vi "LeCroy - Transfer External To Ext Or Ext10.vi"(4 "Trigger Level 2":dbl, 6 "Trigger Level":dbl, 8 "error in (no error)":errorcluster, 10 "Trigger Source With External":u16, 11 "VISA resource name":refnum<visa-resource-name>) -> (0 "error out":errorcluster, 2 "Trigger Source With Ext/Ext10":u16, 3 "VISA resource name out":refnum<visa-resource-name>)   [LabVIEW 8.6]
doc: "This is function which transfer Eternal trigger source to Ext and Ext10. Another trigger source are retained in same state. Transfer External source to Ext and Ext10 is make with compare trigger level. When is trigger level greater than 400 mV (for WaveSurfer 500 mV), than External trigger source is transfer to the Ext10, else is transfer to the Ext."
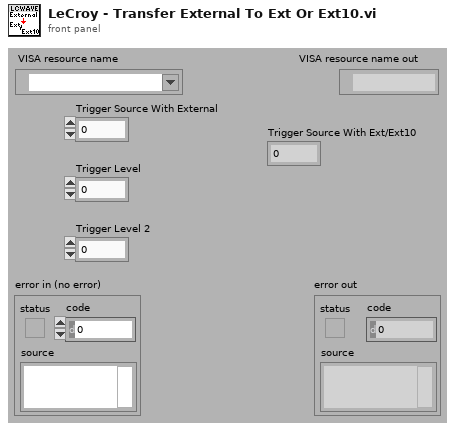
[diagram p1: front panel]
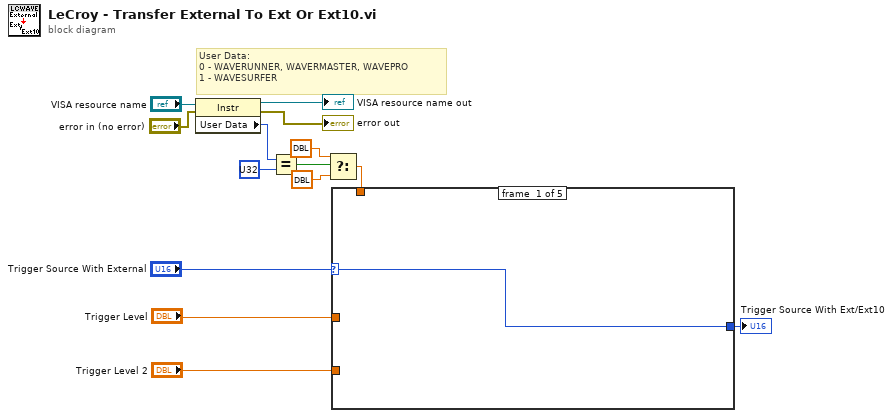
[diagram p0: block diagram]
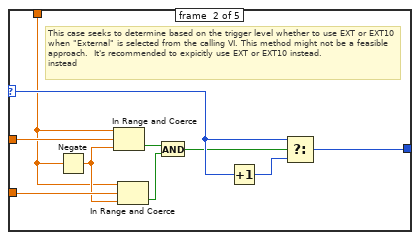
[diagram p2: hidden frame]
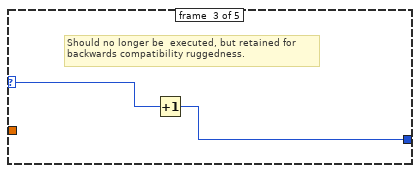
[diagram p3: hidden frame]
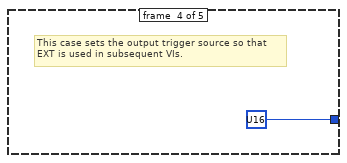
[diagram p4: hidden frame]
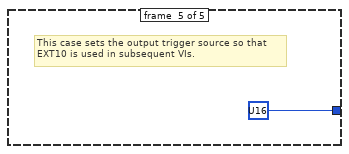
[diagram p5: hidden frame]
diagram:
  # "User Data:\n0 - WAVERUNNER, WAVERMASTER, WAVEPRO\n1 - WAVESURFER"
  n1 = property on="Property Node" class="Instr"(reference="VISA resource name", error in="error in (no error)") -> (reference out=→"VISA resource name out":refnum<visa-resource-name>, error out=→"error out":errorcluster, "User Data"=w6:u32)
  n2 = Equal?(x=w6, y=u32 ?) -> (x = y?=w4:bool)
  n3 = Select(t=dbl ? ("upper limit"), s=w4, f=dbl ? ("upper limit")) -> (s? t:f=w1:dbl)
  n4 = case shown="5" "Trigger Source With External" {
    selector: "Trigger Source With External" -> [w15 w24 w27 _ _]
    tunnel: [w15 w22 w26 u16 ? ("Trigger Source With External") u16 ? ("Trigger Source With External")] -> w12
    tunnel: "Trigger Level" -> [_ w25 _ _ _]
    tunnel: "Trigger Level 2" -> [_ w21 _ _ _]
    tunnel: w1 -> [_ w16 _ _ _]
    frame #0 {
    }
    frame #1 {
      # "This case seeks to determine based on the trigger level whether to use EXT or EXT10 when \"External\" is selected from the calling VI. This method might not be a feasible approach.  It's recommended to expicitly use EXT or EXT10 instead.\ninstead"
      n5 = Negate(x=w16) -> (-x=w17:dbl)
      n6 = In Range and Coerce(upper limit=w16, x=w25, lower limit=w17) -> (In Range?=w20:bool)  [unwired: 1 out]
      n7 = In Range and Coerce(upper limit=w16, x=w21, lower limit=w17) -> (In Range?=w19:bool)  [unwired: 1 out]
      n8 = And(x=w20, y=w19) -> (x .and. y?=w18:bool)
      n9 = Increment(x=w24) -> (x+1=w23:u16)
      n10 = Select(t=w24, s=w18, f=w23) -> (s? t:f=w22:u16)
    }
    frame #2 {
      # "Should no longer be  executed, but retained for \nbackwards compatibility ruggedness."
      n11 = Increment(x=w27) -> (x+1=w26:u16)
    }
    frame #3 {
      # "This case sets the output trigger source so that \nEXT is used in subsequent VIs."
    }
    frame #4 {
      # "This case sets the output trigger source so that \nEXT10 is used in subsequent VIs."
    }
  }
  "Trigger Source With Ext/Ext10" <- w12
